vi "stack_size.vi"() -> ()   [LabVIEW 2013]
panel:
  in  "stack_size":i32=5000
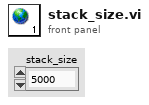
[diagram p1: front panel]
diagram:
